vi "Read Voltage Datas.vi"(9 "length":u32, 10 "buffer":dbl[](array[numeric])=array[4194304 elements], 11 "channel":i8) -> (2 "buffer out":dbl[](array[numeric]), 3 "function return":u32)   [LabVIEW 2021, in "vmmso.lvlib"]
doc: "DLL_API unsigned int WINAPI ReadVoltageDatas(char channel, double* buffer, unsigned int length);"
uses:
  vmmso.lvlib
  vmmso.dll
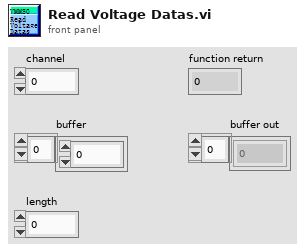
[diagram p1: front panel]
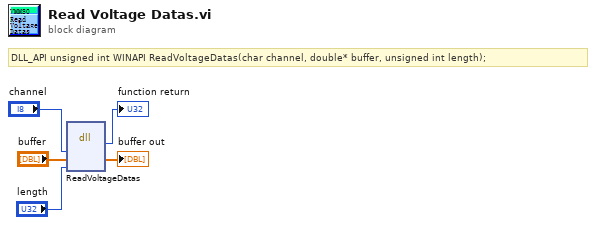
[diagram p0: block diagram]
diagram:
  # "DLL_API unsigned int WINAPI ReadVoltageDatas(char channel, double* buffer, unsigned int length);"
  n1 = dll-call lib="D:/labviewdemo/LabviewDemo 21/vmmso/vmmso.*" fn="ReadVoltageDatas"("channel"="channel", "buffer"="buffer", "length"="length") -> (→"function return":u32, "buffer"=→"buffer out":dbl[])  [unwired: 5 in, 2 out]
